vi "DAQmx Create Channel (AO-Current-Basic).vi"(0 "task in":refnum<k21>, 1 "maximum value":dbl=0.02 format="%0.5f", 2 "minimum value":dbl format="%0.5f", 5 "physical channels":tag, 7 "name to assign":string, 9 "units":i32(ring)=10342 items=["Amps"=10342, "From Custom Scale"=10065], 11 "error in":errorcluster, 12 "custom scale name":tag) -> (4 "task out":refnum<k21>, 15 "error out":errorcluster)   [LabVIEW 2013]
doc: "Creates channel(s) to generate current."
uses:
  C:/Program Files (x86)/National Instruments/LabVIEW 2013/resource/objmgr/daqmx.rc
panel:
  # "output limits"
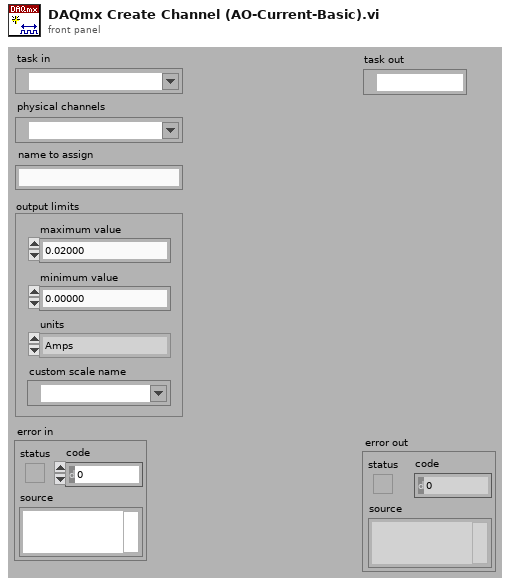
[diagram p1: front panel]
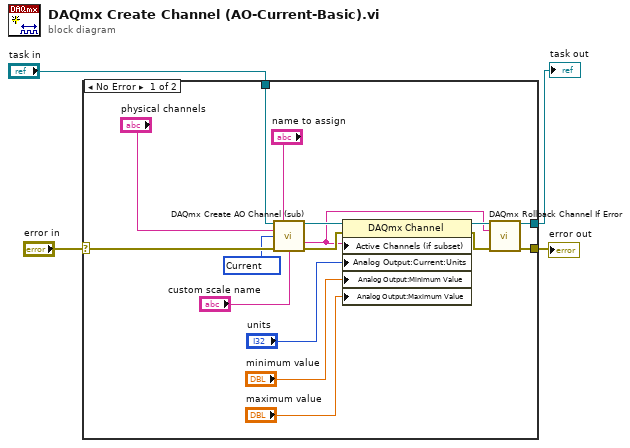
[diagram p0: block diagram]
diagram:
  n1 = case shown="No Error" "error in" {
    selector: "error in" -> [w18 w22]
    tunnel: [w9 w22] -> w4
    tunnel: "task in" -> [w20 w21]
    tunnel: [w7 w21] -> w1
    frame No Error {
      w13 = 10134 items=["Voltage"=10322, "Current"=10134] ("output type")
      n2 = call "DAQmx Create AO Channel (sub).vi"("task in"=w20, "virtual channel name"="name to assign", "physical channel name"="physical channels", "output type"=w13, "error in"=w18, "custom scale"="custom scale name") -> ("task out"=w10:refnum<k21>, "channel names"=w5:string, "error out"=w17:errorcluster)  [unwired: 1 in, 6 out]
      n3 = property class="DAQmx Channel"(reference=w10, error in=w17, "Active Channels (if subset)"=w5, "Analog Output:Current:Units"="units", "Analog Output:Minimum Value"="minimum value", "Analog Output:Maximum Value"="maximum value") -> (reference out=w8:refnum<k21>, error out=w6:errorcluster)
      n4 = call "DAQmx Rollback Channel If Error.vi"("task in"=w8, "channel names"=w5, "error in"=w6) -> ("task out"=w7:refnum<k21>, "error out"=w9:errorcluster)  [unwired: 11 out]
    }
    frame Error {
    }
  }
  "error out" <- w4
  "task out" <- w1
